vi "component center offset.vi"() -> ()   [LabVIEW 2020]
uses:
  <vilib>/Analysis/coordinate.llb/2D Cartesian Coordinate Rotation (Scalar).vi
  <vilib>/Analysis/NI_AALPro.lvlib
panel:
  out "x-y":dbl
  out "Array":dbl[](array[numeric])
  out "tray pos1":dbl[][](array[numeric])
  out "input file":dbl[][](array[numeric])
  out "XY offset":dbl[](array[numeric])
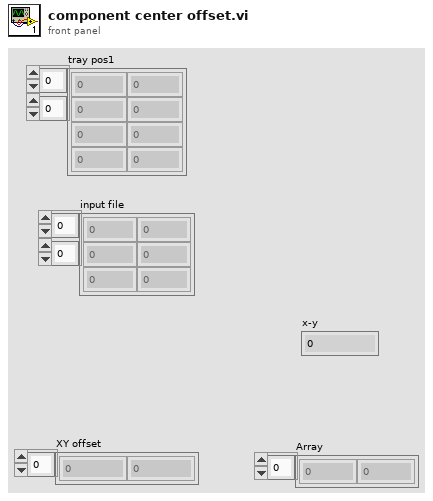
[diagram p1: front panel]
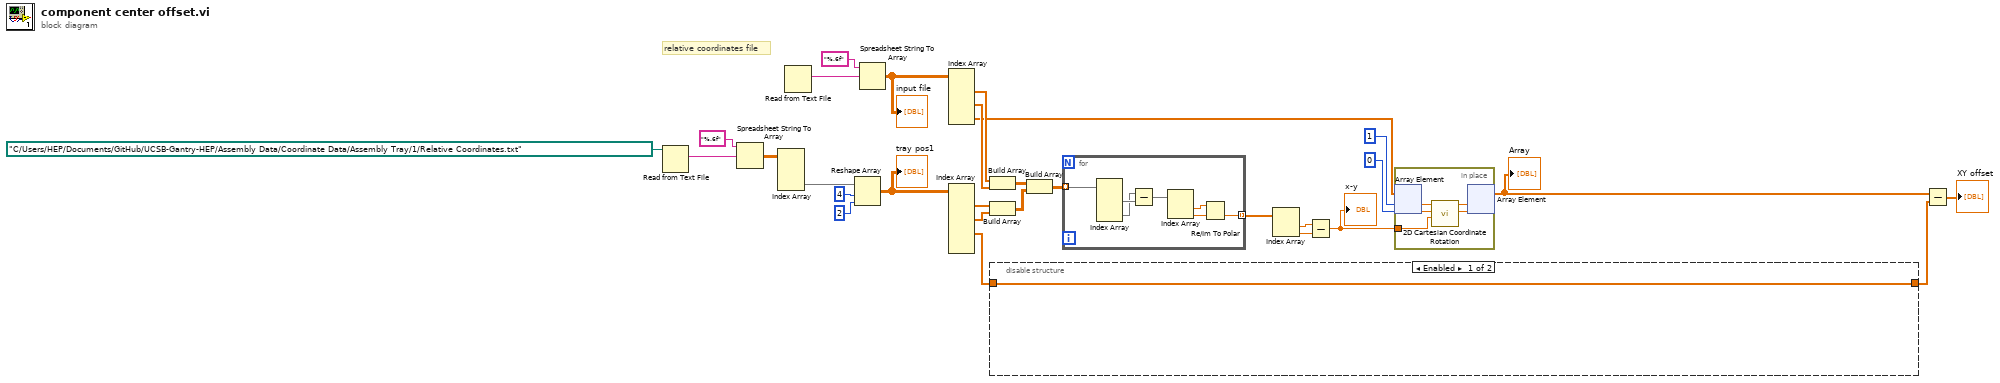
[diagram p0: block diagram]
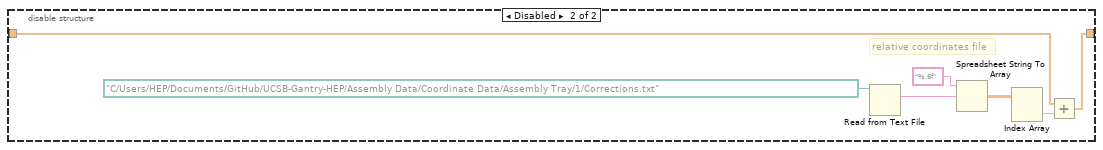
[diagram p2: hidden frame]
diagram:
  # "relative coordinates file"
  n1 = Read from Text File(file (use dialog)=path "C:/Users/HEP/Documents/GitHub/UCSB-Gantry-HEP/Assembly Data/Coordinate Data/Assembly Tray/1/Relative Coordinates.txt") -> (text=w27:string)  [unwired: 3 in, 3 out]
  n2 = Spreadsheet String To Array(format string="%.6f", spreadsheet string=w27) -> (array=w24:dbl[][])  [unwired: 2 in]
  n3 = Index Array(array=w24) -> (element #2=w20:dbl[])  [unwired: 4 in, 1 out]
  n4 = Read from Text File() -> (text=w29:string)  [unwired: 4 in, 3 out]
  n5 = Reshape Array(w20, 4 ("dimension size"), 2 ("dimension size")) -> (w21:dbl[][])
  "tray pos1" <- w21
  n6 = Spreadsheet String To Array(format string="%.6f", spreadsheet string=w29) -> (array=w19:dbl[][])  [unwired: 2 in]
  "input file" <- w19
  n7 = Index Array(array=w19) -> (element #1=w18:dbl[], element #2=w17:dbl[], element #3=w8:dbl[])  [unwired: 6 in]
  n8 = Index Array(array=w21) -> (element #1=w15:dbl[], element #2=w14:dbl[], element #3=w2:dbl[])  [unwired: 8 in, 1 out]
  n9 = Build Array(w18, w17) -> (w16:dbl[][])
  n10 = Build Array(w15, w14) -> (w13:dbl[][])
  n11 = disable-structure shown="Enabled" {
    disable-tunnel: w2 -> [w30 w31]
    disable-tunnel: [w30 w33] -> w1
    frame Enabled {
    }
    frame Disabled {
      # "relative coordinates file"
      n12 = Read from Text File(file (use dialog)=path "C:/Users/HEP/Documents/GitHub/UCSB-Gantry-HEP/Assembly Data/Coordinate Data/Assembly Tray/1/Corrections.txt") -> (text=w37:string)  [unwired: 3 in, 3 out]
      n13 = Spreadsheet String To Array(format string="%.6f", spreadsheet string=w37) -> (array=w34:dbl[][])  [unwired: 2 in]
      n14 = Index Array(array=w34) -> (element=w32:dbl[])  [unwired: 2 in]
      n15 = Add(x=w31, y=w32) -> (x+y=w33:dbl[])
    }
  }
  n16 = Build Array(w16, w13) -> (w12:dbl[][][])
  n17 = for {
    tunnel: w12 -> [w44] mode=indexing
    tunnel: [w38] -> w11 mode=indexing
    n18 = Index Array(array=w44) -> (element #1=w43:dbl[], element #2=w42:dbl[])  [unwired: 4 in]
    n19 = Subtract(x=w42, y=w43) -> (x-y=w41:dbl[])
    n20 = Index Array(array=w41) -> (element #1=w40:dbl, element #2=w39:dbl)  [unwired: 2 in]
    n21 = Re/Im To Polar(2:w39, 3:w40) -> (0:w38:dbl)  [unwired: 1 out]
  }
  n22 = Index Array(array=w11) -> (element #1=w10:dbl, element #2=w9:dbl)  [unwired: 2 in]
  n23 = Subtract(x=w10, y=w9) -> (x-y=w7:dbl)
  "x-y" <- w7
  n24 = in-place {
    in-place-border: w7 -> [w45]
    n25 = in-place-array #1(w8, 1, 0) -> (w49:dbl, w48:dbl)
    n26 = call-poly <vilib>:"2D Cartesian Coordinate Rotation.vi"("theta"=w45, "y"=w48, "x"=w49) -> ("y out"=w46:dbl, "x out"=w47:dbl)  [unwired: 6 in, 1 out]
    n27 = in-place-array #1(w47, w46) -> (w6:dbl[])  [unwired: 2 out]
  }
  "Array" <- w6
  n28 = Subtract(x=w6, y=w1) -> (x-y=→"XY offset":dbl[])
